vi "Target Tracking Controller.vi"(8 "Motor Velocity (deg/s)":dbl, 9 "Filtered Force (N)":dbl, 10 "Force Setpoint (N)":dbl, 11 "Feedback Controller Gains":T1) -> (0 "Motor Velocity Command (deg/s)":dbl, 3 "Error (N)":dbl)   [LabVIEW 2018, in "COBRA Feedback Control Library.lvlib"]
uses:
  COBRA Feedback Control Library.lvlib
  Feedback Controller Gains.ctl
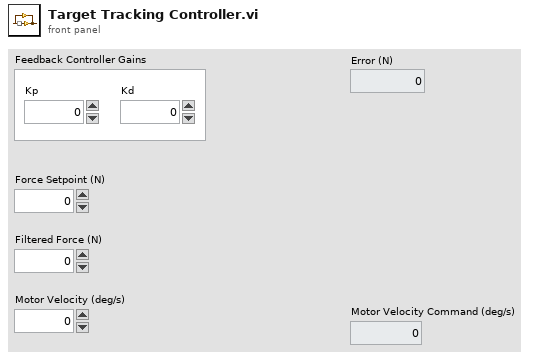
[diagram p1: front panel]
types:
  T1 = typedef "COBRA Feedback Control Library.lvlib/Feedback Controller Gains.ctl" = cluster{"Kp":dbl, "Kd":dbl}
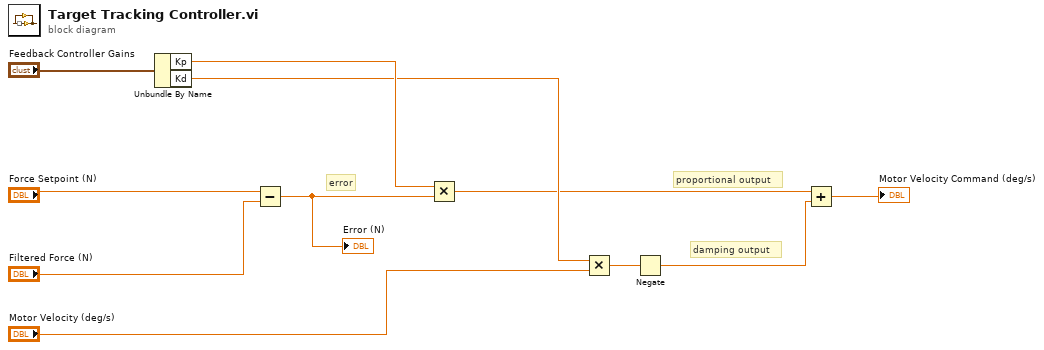
[diagram p0: block diagram]
diagram:
  # "damping output"
  # "proportional output"
  # "error"
  n1 = Unbundle By Name("Feedback Controller Gains") -> ("Kp"=w9:dbl, "Kd"=w8:dbl)
  n2 = Subtract(x="Force Setpoint (N)", y="Filtered Force (N)") -> (x-y=w10:dbl)
  "Error (N)" <- w10
  n3 = Multiply(x=w9, y=w10) -> (x*y=w7:dbl)
  n4 = Multiply(x=w8, y="Motor Velocity (deg/s)") -> (x*y=w6:dbl)
  n5 = Negate(x=w6) -> (-x=w5:dbl)
  n6 = Add(x=w7, y=w5) -> (x+y=→"Motor Velocity Command (deg/s)":dbl)
